vi "get_multiramp_soak_profile_segment_soak_time.vi"(8 "error in (no error)":errorcluster, 10 "Segment number":u8 max=15, 11 "VISA Refnum in":refnum<visa-resource-name>) -> (0 "error out":errorcluster, 2 "Time (s)":dbl max=5999.0, 3 "VISA Refnum out":refnum<visa-resource-name>)   [LabVIEW 2018]
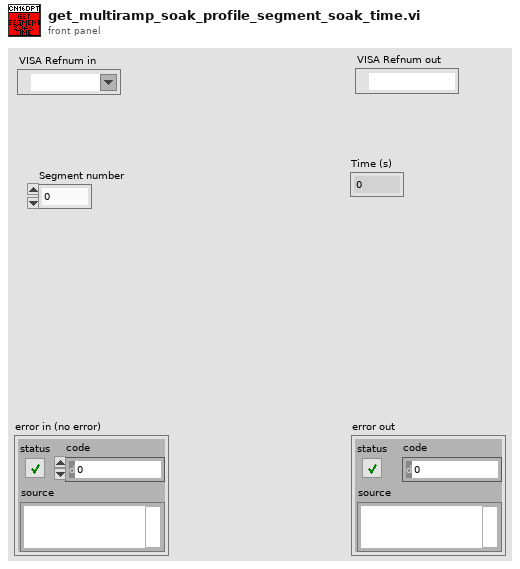
[diagram p1: front panel]
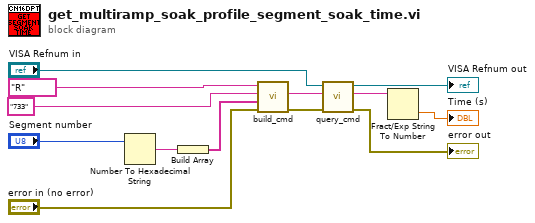
[diagram p0: block diagram]
diagram:
  n1 = Number To Hexadecimal String(2:"Segment number") -> (0:w3:string)  [unwired: 1 in]
  n2 = Build Array(w3) -> (w5:string[])
  n3 = call "build_cmd.vi"("error in (no error)"="error in (no error)", "Parameter list"=w5, "Command ID"="733", "Command class"="R") -> ("error out"=w8:errorcluster, "Command"=w7:string)  [unwired: 6 in]
  n4 = call "query_cmd.vi"("error in (no error)"=w8, "Command"=w7, "VISA resource name"="VISA Refnum in") -> ("error out"=→"error out":errorcluster, "Response"=w2:string, "VISA resource name out"=→"VISA Refnum out":refnum<visa-resource-name>)  [unwired: 6 in]
  n5 = Fract/Exp String To Number(string=w2) -> (number=→"Time (s)":dbl)  [unwired: 3 in, 1 out]
